vi "Read.vi"(11 "NodeInfoValue in":refnum<class "NodeInfoValue.lvclass">) -> (2 "Node Info":T1)   [LabVIEW 2020, in "Vecto.lvlib" / "NodeInfoValue.lvclass"]
uses:
  NodeInfoValue.lvclass
  Task Info.ctl
  Vecto.lvlib
  Node Info.ctl
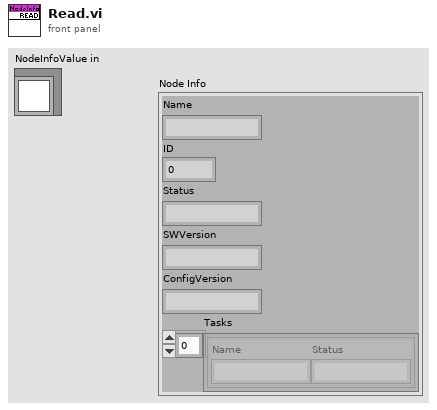
[diagram p1: front panel]
types:
  T1 = typedef "Vecto.lvlib/Node Info.ctl" = cluster{"Name":string, "ID":u32, "Status":string, "SWVersion":string, "ConfigVersion":string, "Tasks":T2[]}
  T2 = typedef "Vecto.lvlib/Task Info.ctl" = cluster{"Name":string, "Status":string}
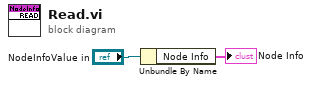
[diagram p0: block diagram]
diagram:
  n1 = Unbundle By Name("NodeInfoValue in") -> ("Node Info"=→"Node Info":T1)
